vi "Open Excel.vi"(0 "excel application in":refnum<k7>, 5 "window state":T1(ring), 7 "display alerts?":bool=TRUE, 11 "error in":errorcluster) -> (4 "excel application out":refnum<k7>, 8 "application already open":bool, 10 "version":string, 15 "error out":errorcluster)   [LabVIEW 2019, in "Simple SysDef API.lvlib"]
uses:
  <userlib>/SimpleSysDef/Simple SysDef API.lvlib
  <vilib>/Utility/NIReport.llb/NI_ReportGenerationCore.lvlib
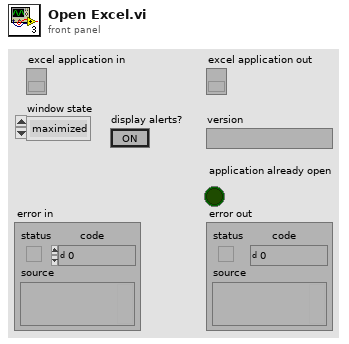
[diagram p1: front panel]
types:
  T1 = enum16{"maximized", "minimized", "normal", "no change"}
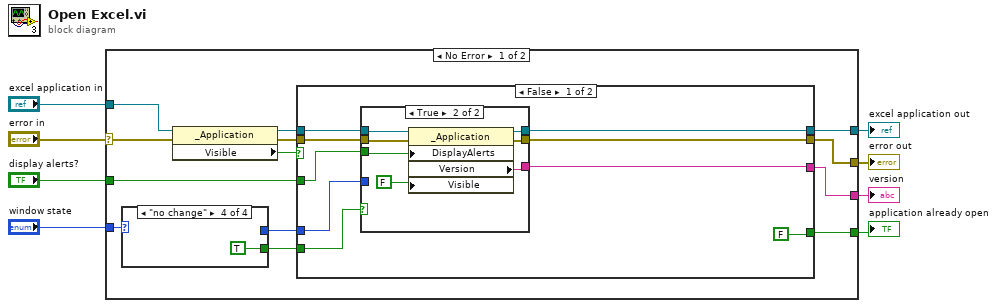
[diagram p0: block diagram]
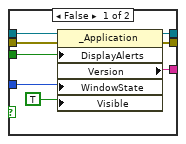
[diagram p2: hidden frame]
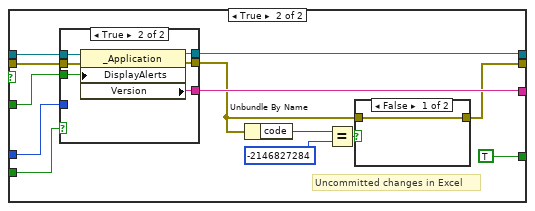
[diagram p3: hidden frame]
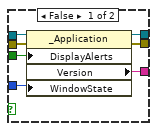
[diagram p4: hidden frame]
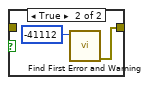
[diagram p5: hidden frame]
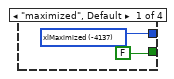
[diagram p6: hidden frame]
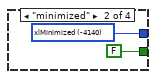
[diagram p7: hidden frame]
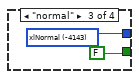
[diagram p8: hidden frame]
diagram:
  n1 = case shown="No Error" "error in" {
    selector: "error in" -> [w9 w83]
    tunnel: "window state" -> [w21 _]
    tunnel: "excel application in" -> [w20 w82]
    tunnel: [w18 w82] -> w6
    tunnel: [w17 w83] -> w5
    tunnel: [w16 _] -> w4
    tunnel: "display alerts?" -> [w13 _]
    tunnel: [w11 _] -> w2
    frame No Error {
      n2 = case shown="\"no change\"" w21 {
        tunnel: [w76 w78 w80 _] -> w19
        tunnel: [FALSE FALSE FALSE TRUE] -> w10
        frame "maximized", Default {
          w76 = -4137 items=["xlMaximized"=-4137, "xlMinimized"=-4140, "xlNormal"=-4143] ("WindowState")
        }
        frame "minimized" {
          w78 = -4140 items=["xlMaximized"=-4137, "xlMinimized"=-4140, "xlNormal"=-4143] ("WindowState")
        }
        frame "normal" {
          w80 = -4143 items=["xlMaximized"=-4137, "xlMinimized"=-4140, "xlNormal"=-4143] ("WindowState")
        }
        frame "no change" {
        }
      }
      n3 = property class="_Application"(reference=w20, error in=w9) -> (reference out=w15:refnum<k7>, error out=w14:errorcluster, "Visible"=w12:bool)
      n4 = case shown="False" w12 {
        tunnel: w19 -> [w24 w54]
        tunnel: [w30 w56] -> w18
        tunnel: [w29 w53] -> w16
        tunnel: [w28 w47] -> w17
        tunnel: w15 -> [w27 w58]
        tunnel: w14 -> [w26 w57]
        tunnel: w13 -> [w25 w52]
        tunnel: [FALSE TRUE] -> w11
        tunnel: w10 -> [w22 w46]
        frame False {
          n5 = case shown="True" w22 {
            tunnel: [w37 w41] -> w30
            tunnel: [w36 w42] -> w29
            tunnel: [w35 w40] -> w28
            tunnel: w27 -> [w34 w43]
            tunnel: w26 -> [w33 w44]
            tunnel: w25 -> [w32 w45]
            tunnel: w24 -> [w31 _]
            frame False {
              n6 = property class="_Application"(reference=w34, error in=w33, "DisplayAlerts"=w32, "WindowState"=w31, "Visible"=TRUE) -> (reference out=w37:refnum<k7>, error out=w35:errorcluster, "Version"=w36:string)
            }
            frame True {
              n7 = property class="_Application"(reference=w43, error in=w44, "DisplayAlerts"=w45, "Visible"=FALSE) -> (reference out=w41:refnum<k7>, error out=w40:errorcluster, "Version"=w42:string)
            }
          }
        }
        frame True {
          # "Uncommitted changes in Excel"
          n8 = case shown="True" w46 {
            tunnel: w58 -> [w59 w71]
            tunnel: w57 -> [w60 w70]
            tunnel: [w61 w69] -> w56
            tunnel: w54 -> [w65 _]
            tunnel: [w63 w68] -> w53
            tunnel: w52 -> [w64 w67]
            tunnel: [w62 w66] -> w48
            frame False {
              n9 = property class="_Application"(reference=w59, error in=w60, "DisplayAlerts"=w64, "WindowState"=w65) -> (reference out=w61:refnum<k7>, error out=w62:errorcluster, "Version"=w63:string)
            }
            frame True {
              n10 = property class="_Application"(reference=w71, error in=w70, "DisplayAlerts"=w67) -> (reference out=w69:refnum<k7>, error out=w66:errorcluster, "Version"=w68:string)
            }
          }
          n11 = Unbundle By Name(w48) -> ("code"=w50:i32)
          n12 = Equal?(x=w50, y=-2146827284) -> (x = y?=w49:bool)
          n13 = case shown="False" w49 {
            tunnel: w48 -> [w72 _]
            tunnel: [w72 w74] -> w47
            frame False {
            }
            frame True {
              n14 = call <vilib>:"Find First Error and Warning.vi"("error code"=-41112 ("code")) -> ("error out"=w74:errorcluster)  [unwired: 1 in, 5 out]
            }
          }
        }
      }
    }
    frame Error {
    }
  }
  "version" <- w4
  "error out" <- w5
  "excel application out" <- w6
  "application already open" <- w2
